vi "VL53L0X_PerformRefSpadManagement.vi"(11 "REV2mDistanceSensorDevRef":T1) -> (1 "isApertureSpads":u8, 2 "refSpadCount":u32, 3 "REV2mDistanceSensorDevRef Out":T1)   [LabVIEW 2019, in "DistanceSensorDriver.lvlib"]
uses:
  DistanceSensorDriver.lvlib
  Typedef/REV2mDistanceSensorDevRef.ctl
  Typedef/Ports.ctl
panel:
  in  "isApertureSpads":u8
  in  "refSpadCount":u32
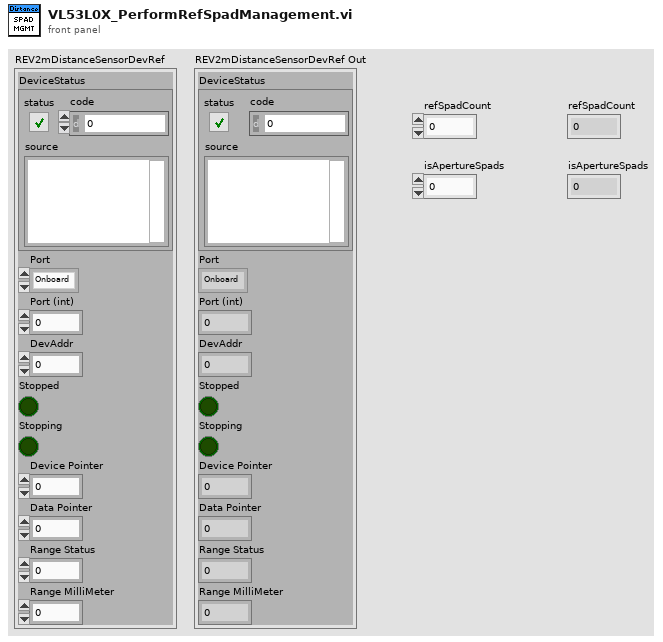
[diagram p1: front panel]
types:
  T1 = typedef "DistanceSensorDriver.lvlib/REV2mDistanceSensorDevRef.ctl" = cluster{"DeviceStatus":errorcluster, "Port":T2, "Port (int)":i32, "DevAddr":i32, "Stopped":bool, "Stopping":bool, "Device Pointer":u64, "Data Pointer":u64, "Range Status":u8, "Range MilliMeter":u16}
  T2 = typedef "DistanceSensorDriver.lvlib/Ports.ctl" = enum32{"Onboard", "MXP"}
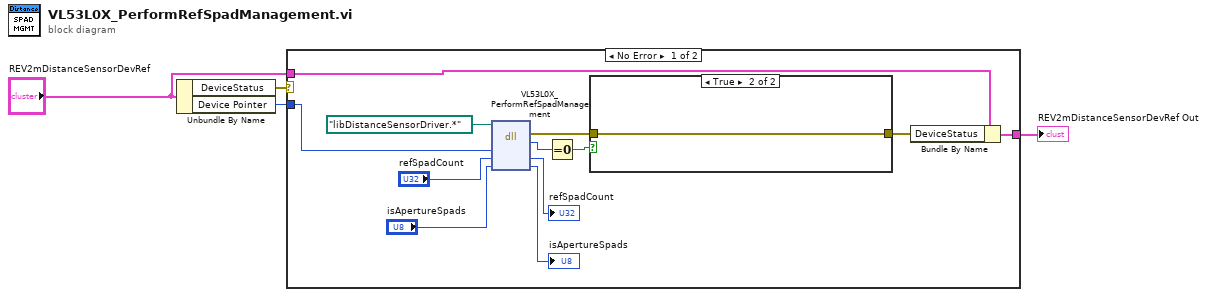
[diagram p0: block diagram]
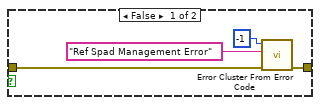
[diagram p2: hidden frame]
diagram:
  n1 = Unbundle By Name("REV2mDistanceSensorDevRef") -> ("DeviceStatus"=w1:errorcluster, "Device Pointer"=w4:u64)
  n2 = case shown="No Error" w1 {
    tunnel: w4 -> [w11 _]
    tunnel: [w10 w22] -> w3
    tunnel: "REV2mDistanceSensorDevRef" -> [w9 w22]
    frame No Error {
      n3 = dll-call lib="?" fn="VL53L0X_PerformRefSpadManagement"(path in=path "libDistanceSensorDriver.*", "Dev"=w11, "refSpadCount"="refSpadCount", "isApertureSpads"="isApertureSpads") -> (error out=w12:errorcluster, "Status"=w13:i32, "refSpadCount"=→"refSpadCount":u32, "isApertureSpads"=→"isApertureSpads":u8)  [unwired: 3 in, 1 out]
      n4 = Equal To 0?(x=w13) -> (x = 0?=w16:bool)
      n5 = case shown="True" w16 {
        tunnel: w12 -> [w17 w21]
        tunnel: [w20 w21] -> w15
        frame False {
          n6 = call <vilib>:"Error Cluster From Error Code.vi"("error in (no error)"=w17, "error message (\"\")"="Ref Spad Management Error" ("error message (\"\")"), "error code (0)"=-1) -> ("error out"=w20:errorcluster)  [unwired: 6 in]
        }
        frame True {
        }
      }
      n7 = Bundle By Name(cluster=w9, "DeviceStatus"=w15) -> (w10:T1)
    }
    frame Error {
    }
  }
  "REV2mDistanceSensorDevRef Out" <- w3
